vi "流程文件XML解析.vi"(5 "简易流程Id":u16(ring), 7 "是否是简易流程":bool, 8 "error in (no error)":errorcluster, 10 "添加的路径":path, 11 "参数簇":T2={"启动参数"=1, "启动模式"=enum."跨度核查", "量程"=enum."低量程"} {"启动参数" items=["总磷"=1, "总氮"=2, "氨氮"=3]}) -> (0 "error out":errorcluster, 3 "数组":T1(array[cluster]) {"port" format="%08x"})   [LabVIEW 2022 SP3, in "斯坦道总磷总氮.lvlib"]
uses:
  <vilib>/xml/Load XML File.vi
  <vilib>/xml/Close Reference(Node).vi
  <resource>/objmgr/DOMUserDefRef.rc
  <vilib>/xml/NI_XML.lvlib
panel:
  in  "数值":i32
  out "字符串":string
  out "大小":i32
  out "XML字符串":string="<?xml version=\"1.0\" encoding=\"ISO-8859-1\"?>\n<bookstore>\n<book ISBN=\"978-0545128285\">\n  <title lang=\"en\">The Tales of Beedle the Bard</title>\n  <author>J. K. Rowling</author>\n  <year>2008</year>\n  <price>12.99</price>\n</book>\n<book ISBN=\"978-0316160209\">\n  <title lang=\"en\">Eclipse</title>\n  <author>Stephenie Meyer</author>\n  <year>2007</year>\n  <price>19.99</price>\n</book>\n<book ISBN=\"978-0316067928\">\n  <title lang=\"en\">Breaking Dawn</title>\n  <author>Stephenie Meyer</author>\n  <year>2008</year>\n  <price>22.99</price>\n</book>\n<book ISBN=\"978-0316017923\">\n  <title lang=\"en\">Outliers: The Story of Success</title>\n  <author>Malcolm Gladwell</author>\n  <year>2008</year>\n  <price>27.99</price>\n</book>\n<book ISBN=\"978-0596007645\">\n  <title lang=\"en\">XML in a Nutshell</title>\n  <author>Elliotte Rusty Harold</author>\n  <author>W. Scott Means</author>\n  <year>2004</year>\n  <price>39.95</price>\n</book>\n</bookstore>"
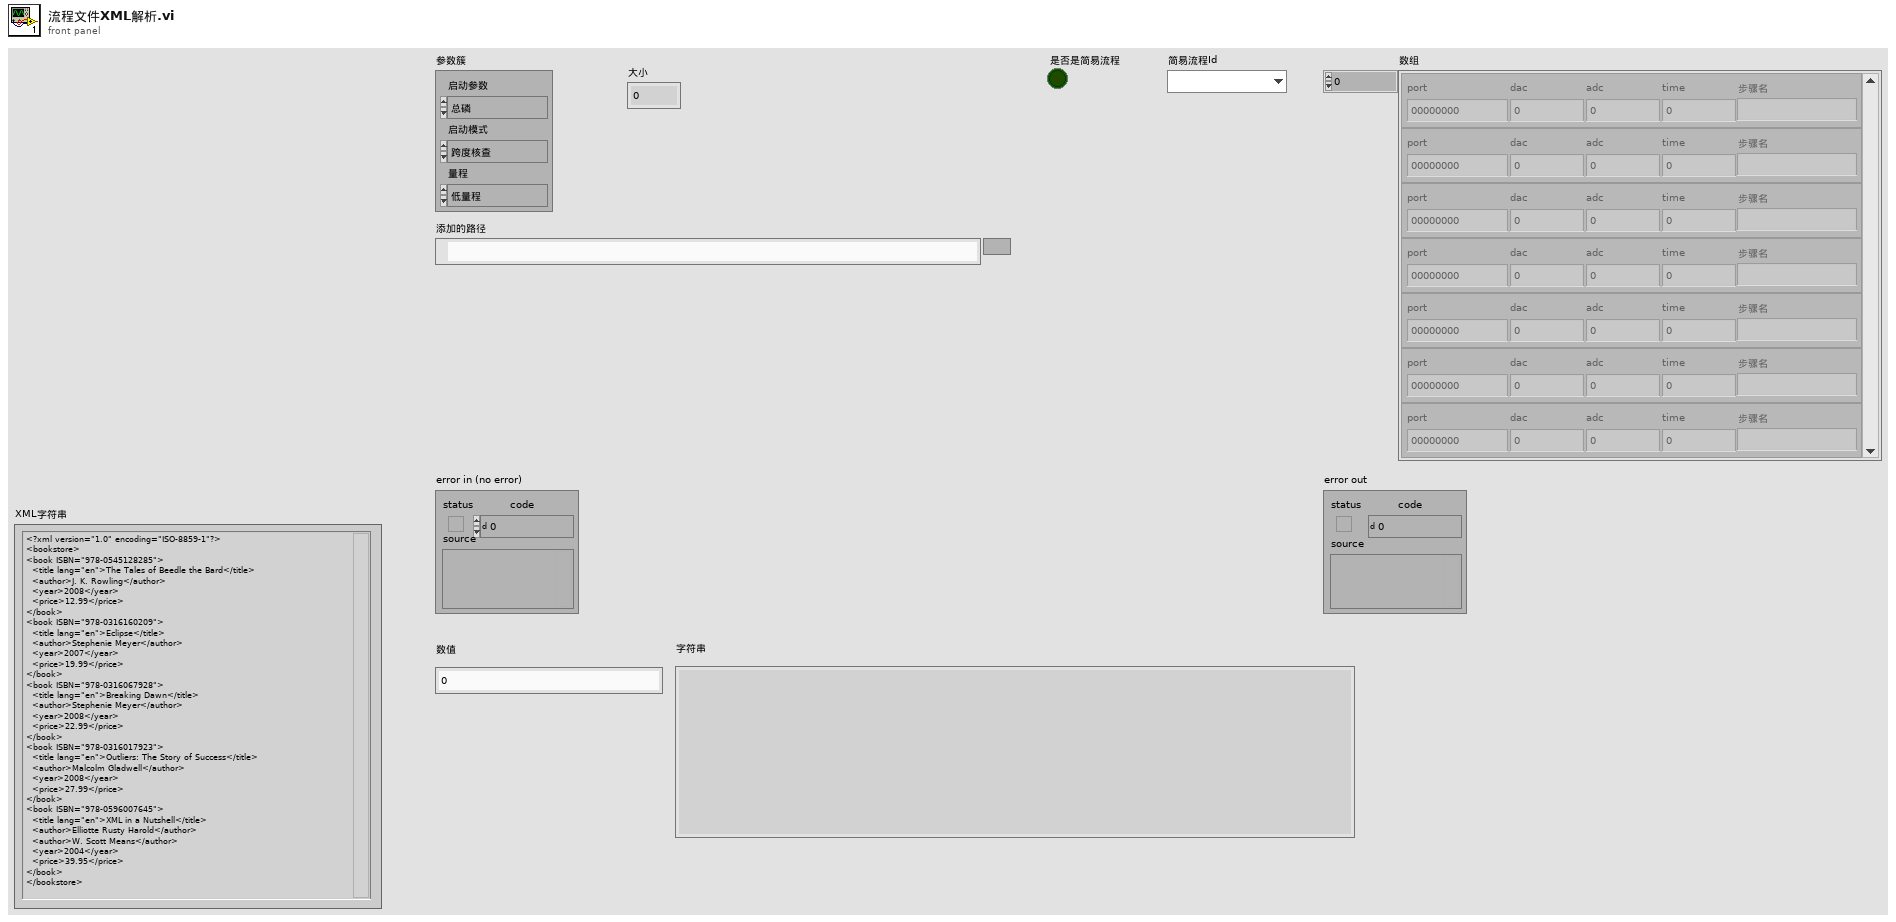
[diagram p1: front panel]
types:
  T1 = cluster{"port":i32, "dac":u8, "adc":u8, "time":u16, "步骤名":string}[]
  T2 = cluster{"启动参数":u16, "启动模式":enum16{"跨度核查", "水样测量", "零点核查", "标样核查", "加标回收", "平行样测试", "空白校准", "标样校准", "空白测试"}, "量程":enum16{"低量程", "高量程"}}
  T3 = enum16{"跨度核查", "水样测量", "零点核查", "标样核查", "加标回收", "平行样测试", "空白校准", "标样校准", "空白测试"}
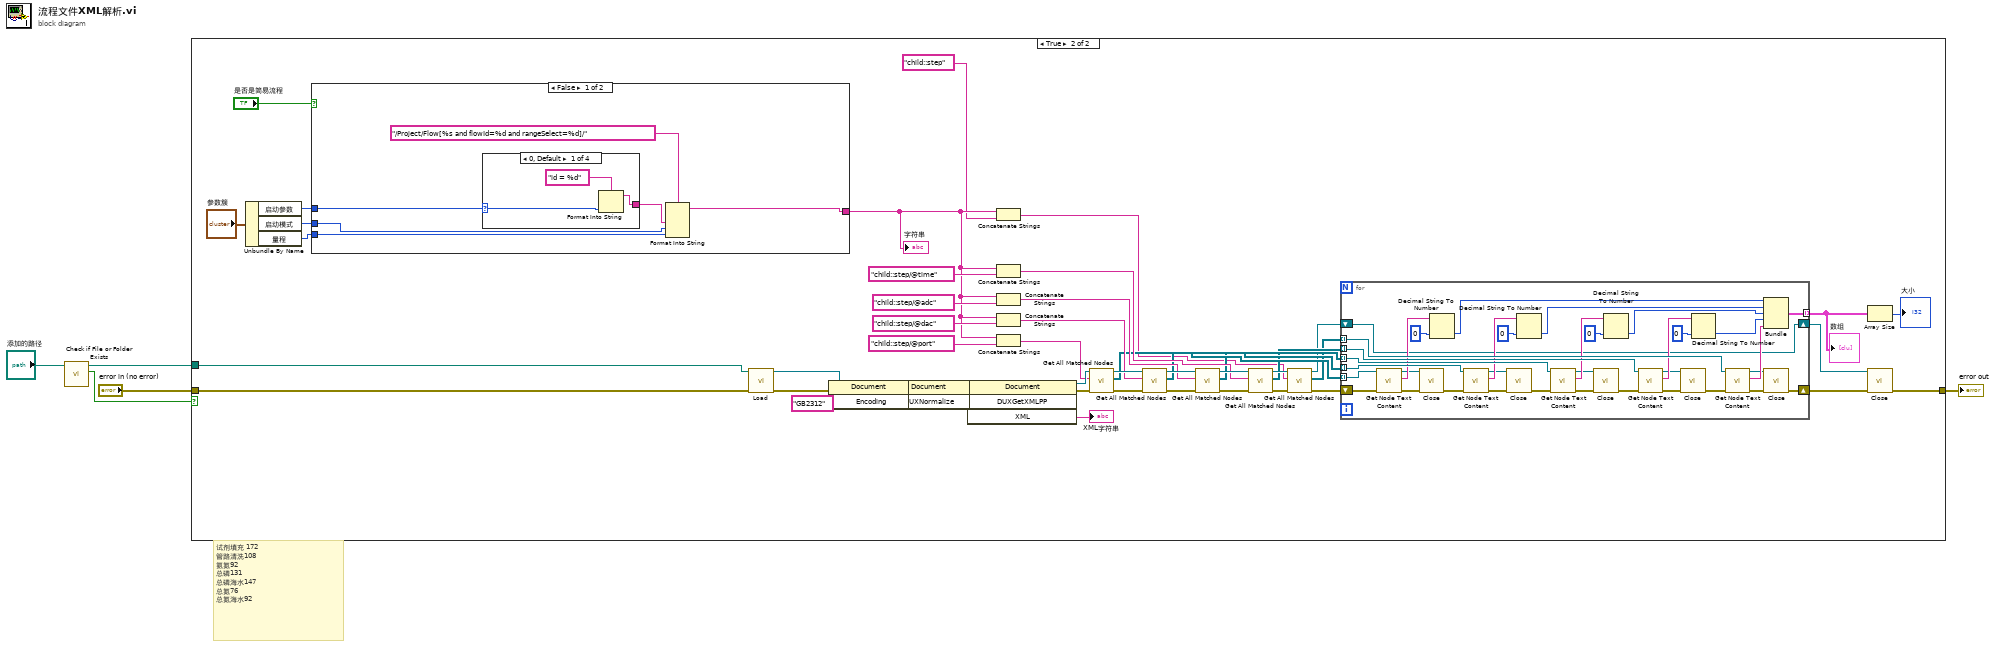
[diagram p0: block diagram]
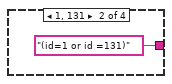
[diagram p3: hidden frame]
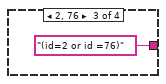
[diagram p4: hidden frame]
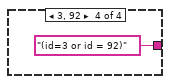
[diagram p5: hidden frame]
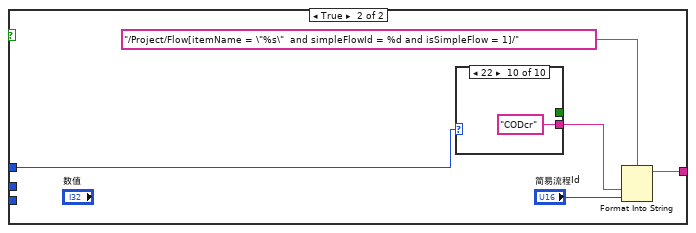
[diagram p6: hidden frame]
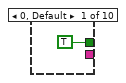
[diagram p7: hidden frame]
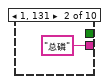
[diagram p8: hidden frame]
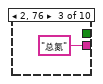
[diagram p9: hidden frame]
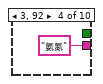
[diagram p10: hidden frame]
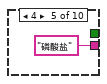
[diagram p11: hidden frame]
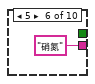
[diagram p12: hidden frame]
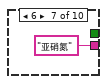
[diagram p13: hidden frame]
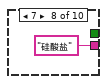
[diagram p14: hidden frame]
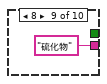
[diagram p15: hidden frame]
diagram:
  # "试剂填充 172 \n管路清洗108\n氨氮92\n总磷131\n总磷海水147\n总氮76\n总氮海水92"
  n1 = call <vilib>:"Check if File or Folder Exists.vi"("path"="添加的路径") -> ("file or folder exists?"=w3:bool, "dup path"=w4:path)  [unwired: 8 in, 1 out]
  n2 = case shown="True" w3 {
    tunnel: w4 -> [_ w41]
    tunnel: "error in (no error)" -> [w6 w9]
    tunnel: [w6 w7] -> w1
    frame False {
    }
    frame True {
      n3 = Unbundle By Name("参数簇") -> ("启动参数"=w42:u16, "启动模式"=w45:T3, "量程"=w44:enum16{"低量程", "高量程"})
      n4 = case shown="False" "是否是简易流程" {
        tunnel: w45 -> [w59 _]
        tunnel: w44 -> [w58 _]
        tunnel: w42 -> [w57 w68]
        tunnel: [w55 w70] -> w23
        frame False {
          n5 = case shown="0, Default" w57 {
            selector: w57 -> [w62 _ _ _]
            tunnel: [w61 "(id=1 or id =131)" ("输入 4") "(id=2 or id =76)" ("输入 4") "(id=3 or id = 92)" ("输入 4")] -> w56
            frame 0, Default {
              n6 = Format Into String(format string="id = %d" ("格式字符串"), w62) -> (resulting string=w61:string)  [unwired: 2 in, 1 out]
            }
            frame 1, 131 {
            }
            frame 2, 76 {
            }
            frame 3, 92 {
            }
          }
          n7 = Format Into String(format string="/Project/Flow[%s and flowId=%d and rangeSelect=%d]/" ("XPath expression"), w56, w59, w58) -> (resulting string=w55:string)  [unwired: 2 in, 1 out]
        }
        frame True {
          n8 = case shown="22" w68 {
            tunnel: [_ "总磷" ("table输入") "总氮" ("table输入") "氨氮" ("table输入") "磷酸盐" ("table输入") "硝氮" ("table输入") "亚硝氮" ("table输入") "硅酸盐" ("table输入") "硫化物" ("table输入") "CODcr" ("table输入")] -> w67
            tunnel: [TRUE _ _ _ _ _ _ _ _ _] -> _
            frame 0, Default {
            }
            frame 1, 131 {
            }
            frame 2, 76 {
            }
            frame 3, 92 {
            }
            frame 4 {
            }
            frame 5 {
            }
            frame 6 {
            }
            frame 7 {
            }
            frame 8 {
            }
            frame 22 {
            }
          }
          n9 = Format Into String(format string="/Project/Flow[itemName = \"%s\"  and simpleFlowId = %d and isSimpleFlow = 1]/" ("XPath expression"), w67, "简易流程Id") -> (resulting string=w70:string)  [unwired: 2 in, 1 out]
        }
      }
      "字符串" <- w23
      n10 = call-poly <vilib>:"Load.vi"("path to XML document"=w41, "error in (no error)"=w9) -> ("DOM document out"=w52:refnum<k20>, "error out"=w51:errorcluster)  [unwired: 11 in, 1 out]
      n11 = property on="属性节点" class="Document"(reference=w52, error in=w51, "Encoding"="GB2312" ("文档编码")) -> (reference out=w50:refnum<k20>, error out=w49:errorcluster)
      n12 = invoke on="Invoke Node" class="Document" method="DUXNormalize"(reference=w50, error in=w49) -> (reference out=w47:refnum<k20>, error out=w48:errorcluster)  [unwired: 1 in, 1 out]
      n13 = invoke on="Invoke Node" class="Document" method="DUXGetXMLPP"(reference=w47, error in=w48) -> (reference out=w40:refnum<k20>, error out=w14:errorcluster, "XML"=→"XML字符串":string)  [unwired: 2 in, 1 out]
      n14 = Concatenate Strings(w23, "child::step" ("输入 4")) -> (w16:string)
      n15 = Concatenate Strings(w23, "child::step/@time" ("输入 4")) -> (w25:string)
      n16 = Concatenate Strings(w23, "child::step/@adc" ("输入 4")) -> (w27:string)
      n17 = Concatenate Strings(w23, "child::step/@dac" ("输入 4")) -> (w29:string)
      n18 = Concatenate Strings(w23, "child::step/@port" ("输入 4")) -> (w39:string)
      n19 = call <vilib>:"Get All Matched Nodes.vi"("error in (no error)"=w14, "XPath expression"=w39, "node in"=w40) -> ("error out"=w36:errorcluster, "node result array"=w21:refnum<k20>[], "node out"=w37:refnum<k20>)  [unwired: 6 in]
      n20 = call <vilib>:"Get All Matched Nodes.vi"("error in (no error)"=w36, "XPath expression"=w29, "node in"=w37) -> ("error out"=w35:errorcluster, "node result array"=w20:refnum<k20>[], "node out"=w34:refnum<k20>)  [unwired: 6 in]
      n21 = call <vilib>:"Get All Matched Nodes.vi"("error in (no error)"=w35, "XPath expression"=w27, "node in"=w34) -> ("error out"=w33:errorcluster, "node result array"=w19:refnum<k20>[], "node out"=w32:refnum<k20>)  [unwired: 6 in]
      n22 = call <vilib>:"Get All Matched Nodes.vi"("error in (no error)"=w33, "XPath expression"=w25, "node in"=w32) -> ("error out"=w31:errorcluster, "node result array"=w18:refnum<k20>[], "node out"=w30:refnum<k20>)  [unwired: 6 in]
      n23 = call <vilib>:"Get All Matched Nodes.vi"("error in (no error)"=w31, "XPath expression"=w16, "node in"=w30) -> ("error out"=w15:errorcluster, "node result array"=w17:refnum<k20>[], "node out"=w8:refnum<k20>)  [unwired: 6 in]
      n24 = for {
        tunnel: w21 -> [w117] mode=indexing
        tunnel: w20 -> [w116] mode=indexing
        tunnel: w19 -> [w115] mode=indexing
        tunnel: w18 -> [w114] mode=indexing
        tunnel: w17 -> [w113] mode=indexing
        tunnel: [w99] -> w11 mode=indexing
        shift-right: [w97] -> w12
        shift-left: w8 -> [w97]
        shift-right: [w82] -> w13
        shift-left: w15 -> [w98]
        n25 = call <vilib>:"Get Node Text Content.vi"("error in (no error)"=w98, "node in"=w117) -> ("error out"=w96:errorcluster, "node text"=w112:string, "node out"=w95:refnum<k20>)  [unwired: 7 in]
        n26 = call-poly <vilib>:"Close.vi"("error in (no error)"=w96, "node"=w95) -> ("error out"=w86:errorcluster)  [unwired: 7 out]
        n27 = Decimal String To Number(string=w112, default (0L)=0 ("默认(0 I32)")) -> (number=w104:i32)  [unwired: 1 in, 1 out]
        n28 = call <vilib>:"Get Node Text Content.vi"("error in (no error)"=w86, "node in"=w116) -> ("error out"=w93:errorcluster, "node text"=w109:string, "node out"=w94:refnum<k20>)  [unwired: 7 in]
        n29 = call-poly <vilib>:"Close.vi"("error in (no error)"=w93, "node"=w94) -> ("error out"=w85:errorcluster)  [unwired: 7 out]
        n30 = Decimal String To Number(string=w109, default (0L)=u8 0 ("默认(0 I32)")) -> (number=w103:u8)  [unwired: 1 in, 1 out]
        n31 = call <vilib>:"Get Node Text Content.vi"("error in (no error)"=w85, "node in"=w115) -> ("error out"=w89:errorcluster, "node text"=w106:string, "node out"=w92:refnum<k20>)  [unwired: 7 in]
        n32 = call-poly <vilib>:"Close.vi"("error in (no error)"=w89, "node"=w92) -> ("error out"=w84:errorcluster)  [unwired: 7 out]
        n33 = Decimal String To Number(string=w106, default (0L)=u8 0 ("默认(0 I32)")) -> (number=w102:u8)  [unwired: 1 in, 1 out]
        n34 = call <vilib>:"Get Node Text Content.vi"("error in (no error)"=w84, "node in"=w114) -> ("error out"=w88:errorcluster, "node text"=w105:string, "node out"=w91:refnum<k20>)  [unwired: 7 in]
        n35 = call-poly <vilib>:"Close.vi"("error in (no error)"=w88, "node"=w91) -> ("error out"=w83:errorcluster)  [unwired: 7 out]
        n36 = Decimal String To Number(string=w105, default (0L)=u16 0 ("默认(0 I32)")) -> (number=w101:u16)  [unwired: 1 in, 1 out]
        n37 = call <vilib>:"Get Node Text Content.vi"("error in (no error)"=w83, "node in"=w113) -> ("error out"=w87:errorcluster, "node text"=w100:string, "node out"=w90:refnum<k20>)  [unwired: 7 in]
        n38 = Bundle(w104, w103, w102, w101, "node text"=w100) -> (w99:cluster{i32, u8, u8, u16, "node text":string})  [unwired: 1 in]
        n39 = call-poly <vilib>:"Close.vi"("error in (no error)"=w87, "node"=w90) -> ("error out"=w82:errorcluster)  [unwired: 7 out]
      }
      "数组" <- w11
      n40 = Array Size(array=w11) -> (size(s)=→"大小":i32)
      n41 = call-poly <vilib>:"Close.vi"("error in (no error)"=w13, "node"=w12) -> ("error out"=w7:errorcluster)  [unwired: 7 out]
    }
  }
  "error out" <- w1
